vi "ComplexNumbers.vi"(4 "Array 2D":cdb[][](array[numeric])=[[1.0+4.0i, 53.0+87.0i, 11.0+71.0i], [33.0+52.0i, 71.0+82.0i, 55.0+89.0i]], 6 "Array 2":T1(array[cluster])=[{"Numeric"=5.0-89.0i, "Numeric 2"=-12.0+19.0i, "Array"=[79.0+90.0i, 122.0-578.0i, 22.0+12.0i]}], 8 "Complex Waveform":waveform(cdb)={"t0"=timestamp(3382639562.007699 s since 1904-01-01), "dt"=1.0, "Y"=[4.0+3.0i, 5.0+2.0i, 6.0+1.0i, 7.0+0.0i]}, 9 "Array":csg[](array[numeric])=[11.0+33.0i, 22.0+44.0i, 55.0+77.0i, 66.0+88.0i], 10 "Cluster":cluster{"Numeric":cdb, "Numeric 2":cxt}={"Numeric"=121.0+147.0i, "Numeric 2"=123.0+456.0i}, 11 "Numeric":cdb=1.0+34.0i) -> ()   [LabVIEW 2010]
panel:
  in  "stop":bool
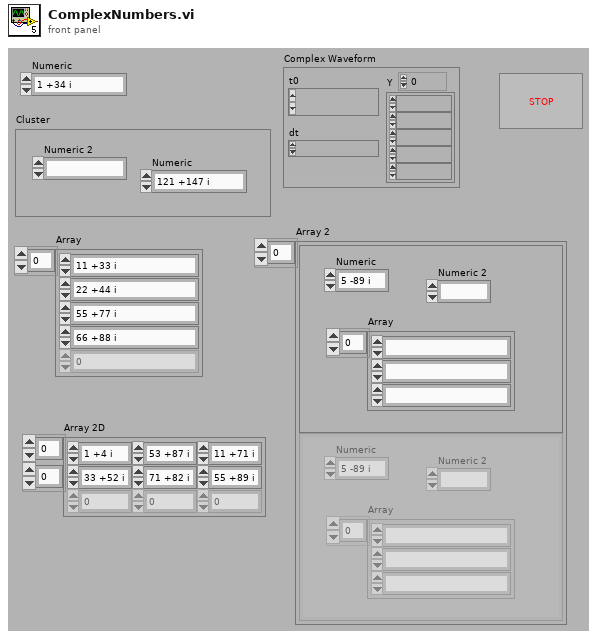
[diagram p1: front panel]
types:
  T1 = cluster{"Numeric":csg, "Numeric 2":cxt, "Array":cdb[]}[]
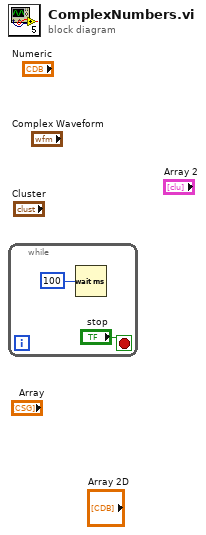
[diagram p0: block diagram]
diagram:
  n1 = while {
    stop <- "stop" stop-if-true
    n2 = Wait (ms)(milliseconds to wait=u32 100) -> ()  [unwired: 1 out]
  }
